vi "ziGetValueString.vi"(3 "error in":errorcluster, 4 "Path":string, 5 "Handle In":T1 {"Handle" format="0x%08x"; "Conn" format="0x%08x"}) -> (0 "error out":errorcluster, 1 "Value":string, 2 "Handle Out":T1 {"Handle" format="0x%08x"; "Conn" format="0x%08x"})   [LabVIEW 2009, in "Zurich Instruments LabOne.lvlib"]
doc: "This vi retrieves the value of the node node specified by <b>Path</b> as a string <b>value</b>. The vi returns the value of the node first found if more than one node is available (a wildcard is used in <b>Path</b>). This function is only applicable to nodes that contain strings."
uses:
  <instrlib>/Zurich Instruments LabOne/Zurich Instruments LabOne.lvlib
  <instrlib>/Zurich Instruments LabOne/Public/ziTypeHandle.ctl
  <instrlib>/Zurich Instruments LabOne/Private/ziLV32.dll
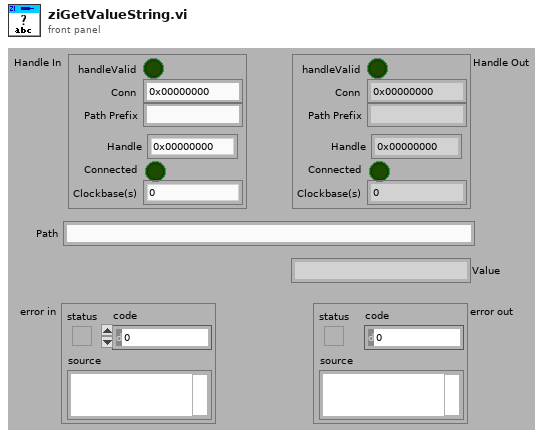
[diagram p1: front panel]
types:
  T1 = typedef "Zurich Instruments LabOne.lvlib/ziTypeHandle.ctl" = cluster{"handleValid":bool, "Conn":u64, "Path Prefix":string, "Handle":u64, "Connected":bool, "Clockbase(s)":dbl}
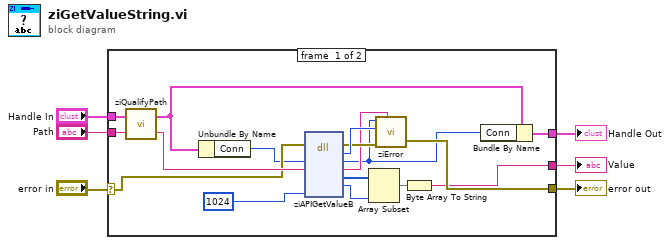
[diagram p0: block diagram]
diagram:
  n1 = case shown="No Error" "error in" {
    selector: "error in" -> [w10 w25]
    tunnel: [w21 w25] -> w6
    tunnel: [w20 w24] -> w5
    tunnel: "Handle In" -> [w19 w24]
    tunnel: "Path" -> [w17 _]
    tunnel: [w11 _] -> w2
    frame #0 {
      n2 = call <instrlib>:"ziQualifyPath.vi"("Path In"=w17, "Handle In"=w19) -> ("Path Out"=w16:string, "Handle Out"=w18:T1)
      n3 = Unbundle By Name(w18) -> ("Conn"=w8:u64)
      n4 = dll-call lib="C:/Program Files (x86)/National Instruments/LabVIEW 2009/instr.lib/Zurich Instruments LabOne/Private/ziLV*.*" fn="ziAPIGetValueB"(error in=w10, "Conn"=w8, "Path"=w16, "MaxLen"=1024) -> (error out=w22:errorcluster, "return type"=w23:u32, "Conn"=w7:u64, "Path"=w9:string, "Buffer"=w14:i8[], "Len"=w13:i32)  [unwired: 2 in, 4 out]
      n5 = Array Subset(array=w14, length=w13) -> (w12:i8[])  [unwired: 1 in]
      n6 = call <instrlib>:"ziError.vi"("Conn"=w7, "ziErrorCode"=w23, "Error In"=w22, "Annotation"=w9) -> ("Error Out"=w21:errorcluster)  [unwired: 2 in]
      n7 = Byte Array To String(unsigned byte array=w12) -> (string=w11:string)
      n8 = Bundle By Name(cluster=w18, "Conn"=w7) -> (w20:T1)
    }
    frame #1 {
    }
  }
  "Handle Out" <- w5
  "error out" <- w6
  "Value" <- w2
